vi "Get relay numbers.vi"(11 "Variant":string) -> (2 "DUT2":T1, 3 "DUT1":T1)   [LabVIEW 2023]
uses:
  <vilib>/Utility/config.llb/Read Key (I32).vi
  <vilib>/Utility/config.llb/NI_LVConfig.lvlib
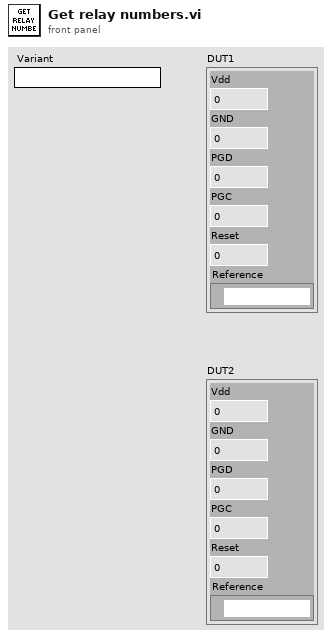
[diagram p1: front panel]
types:
  T1 = cluster{"Vdd":i32, "GND":i32, "PGD":i32, "PGC":i32, "Reset":i32, "Reference":refnum<visa-resource-name>}
  T2 = typedef "NI_LVConfig.lvlib/Config Data RefNum.ctl" = refnum<k1>
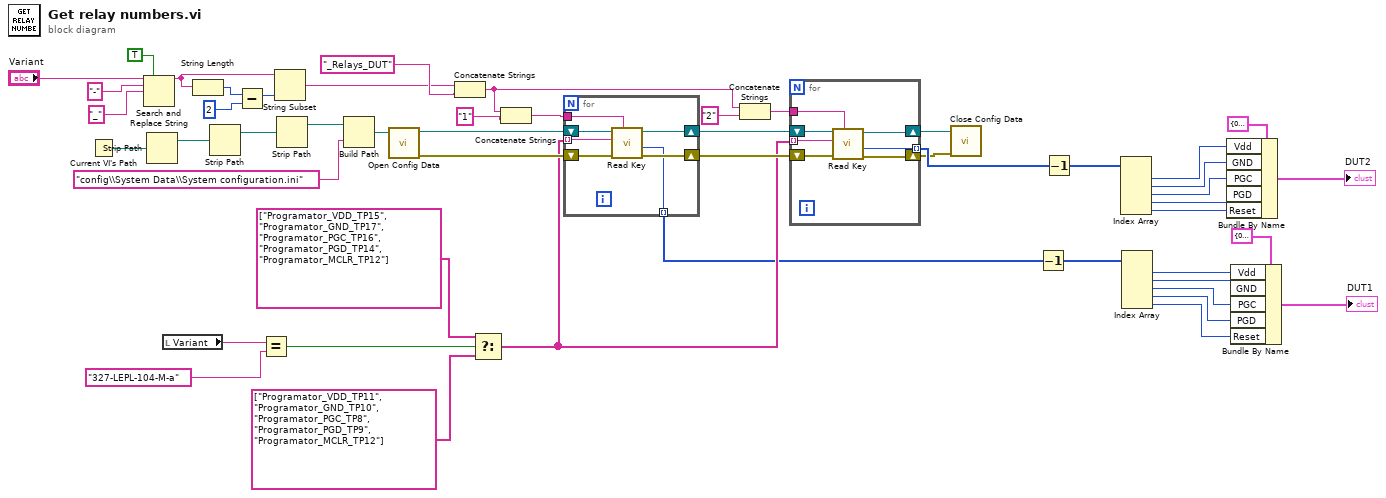
[diagram p0: block diagram]
diagram:
  n1 = Current VI's Path() -> (path=w50:path)
  n2 = Search and Replace String(replace all?=TRUE ("replace all? (F)"), input string="Variant", search string="-" ("replace string (\"\")"), replace string="_" ("replace string (\"\")")) -> (result string=w6:string)  [unwired: 4 in, 3 out]
  n3 = Strip Path(path=w50) -> (stripped path=w49:path)  [unwired: 1 out]
  n4 = local read "Variant"() -> (w29:string)
  n5 = String Length(string=w6) -> (length=w5:i32)
  n6 = Strip Path(path=w49) -> (stripped path=w48:path)  [unwired: 1 out]
  n7 = Subtract(x=w5, y=2) -> (x-y=w3:i32)
  n8 = Equal?(x=w29, y="327-LEPL-104-M-a") -> (x = y?=w27:bool)
  n9 = String Subset(string=w6, length (rest)=w3) -> (substring=w7:string)  [unwired: 1 in]
  n10 = Strip Path(path=w48) -> (stripped path=w47:path)  [unwired: 1 out]
  n11 = Build Path(base path=w47, name or relative path="config\\System Data\\System configuration.ini") -> (appended path=w51:path)
  n12 = call <vilib>:"Open Config Data.vi"("configuration file path"=w51) -> ("error out"=w30:errorcluster, "refnum"=w43:T2)  [unwired: 8 in, 1 out]
  n13 = Concatenate Strings(w7, "_Relays_DUT" ("string")) -> (w35:string)
  n14 = Select(t=string[] ["Programator_VDD_TP15", "Programator_GND_TP17", "Programator_PGC_TP16", "Programator_PGD_TP14", "Programator_MCLR_TP12"], s=w27, f=string[] ["Programator_VDD_TP11", "Programator_GND_TP10", "Programator_PGC_TP8", "Programator_PGD_TP9", "Programator_MCLR_TP12"]) -> (s? t:f=w24:string[])
  n15 = Concatenate Strings(w35, "1" ("string")) -> (w36:string)
  n16 = for {
    tunnel: w36 -> [w57]
    shift-right: [w56] -> w32
    shift-left: w43 -> [w58]
    shift-right: [w55] -> w31
    shift-left: w30 -> [w54]
    tunnel: w24 -> [w53] mode=indexing
    tunnel: [w52] -> w23 mode=indexing
    n17 = call-poly <vilib>:"Read Key.vi"("section"=w57, "error in (no error)"=w54, "key"=w53, "refnum"=w58) -> ("error out"=w55:errorcluster, "value"=w52:i32, "refnum out"=w56:T2)  [unwired: 4 in, 1 out]
  }
  n18 = Concatenate Strings(w35, "2" ("string")) -> (w33:string)
  n19 = for {
    tunnel: w33 -> [w65]
    shift-right: [w62] -> w8
    shift-left: w32 -> [w64]
    shift-right: [w61] -> w9
    shift-left: w31 -> [w63]
    tunnel: w24 -> [w60] mode=indexing
    tunnel: [w59] -> w17 mode=indexing
    n20 = call-poly <vilib>:"Read Key.vi"("section"=w65, "error in (no error)"=w63, "key"=w60, "refnum"=w64) -> ("error out"=w61:errorcluster, "value"=w59:i32, "refnum out"=w62:T2)  [unwired: 4 in, 1 out]
  }
  n21 = call <vilib>:"Close Config Data.vi"("error in (no error)"=w9, "refnum"=w8) -> ()  [unwired: 8 in, 2 out]
  n22 = Decrement(x=w23) -> (x-1=w1:i32[])
  n23 = Decrement(x=w17) -> (x-1=w2:i32[])
  n24 = Index Array(array=w2) -> (element #1=w16:i32, element #2=w15:i32, element #3=w14:i32, element #4=w13:i32, element #5=w12:i32)  [unwired: 5 in]
  n25 = Index Array(array=w1) -> (element #1=w22:i32, element #2=w21:i32, element #3=w20:i32, element #4=w19:i32, element #5=w18:i32)  [unwired: 5 in]
  n26 = Bundle By Name(cluster=T1 {"Vdd"=0, "GND"=0, "PGD"=0, "PGC"=0, "Reset"=0, "Reference"=""} ("Releji DUT1"), "Vdd"=w16, "GND"=w15, "PGC"=w14, "PGD"=w13, "Reset"=w12) -> (→"DUT2":T1)
  n27 = Bundle By Name(cluster=T1 {"Vdd"=0, "GND"=0, "PGD"=0, "PGC"=0, "Reset"=0, "Reference"=""} ("Releji DUT1"), "Vdd"=w22, "GND"=w21, "PGC"=w20, "PGD"=w19, "Reset"=w18) -> (→"DUT1":T1)
